vi "Large int-multiplty a and b.vi"(8 "error in (no error)":errorcluster, 10 "b = Large int (decimal)":string, 11 "a = Large int (decimal)":string) -> (0 "error out":errorcluster, 2 "T = the inputs are integers (contain only digits)":bool, 3 "c = a x b":string)   [LabVIEW 2021, in "Numeric Utilities.lvlib"]
uses:
  Numeric Utilities.lvlib
panel:
  out "longer integer":string
  out "shorter integer":string
  out "Loop iteration":i32
  # "Development\ncontrols/indicators useful for development and testing, but which are not outputs of the VI"
  # "Input\nInputs to the VI"
  # "Output\nOutputs of the VI"
  # "Description\n\nBlank VI with error handling case. \n\nSummarize the use of this VI in this space."
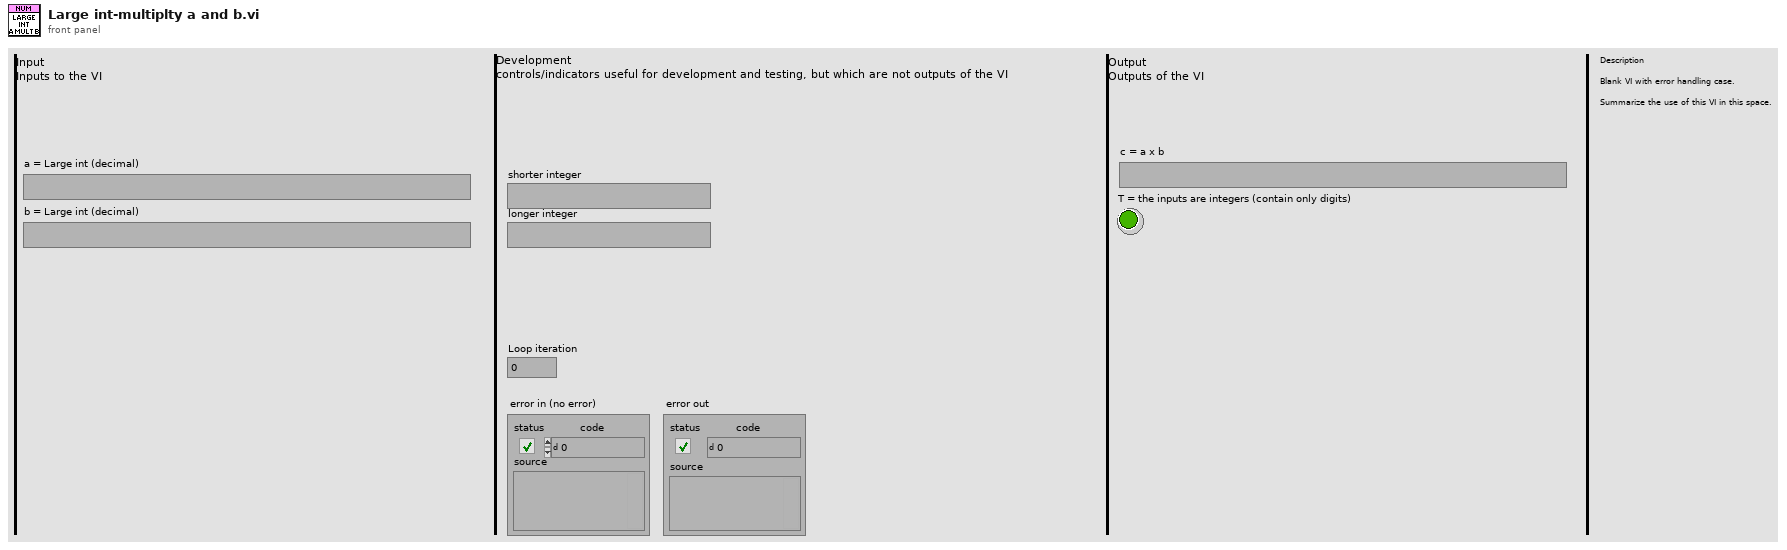
[diagram p1: front panel]
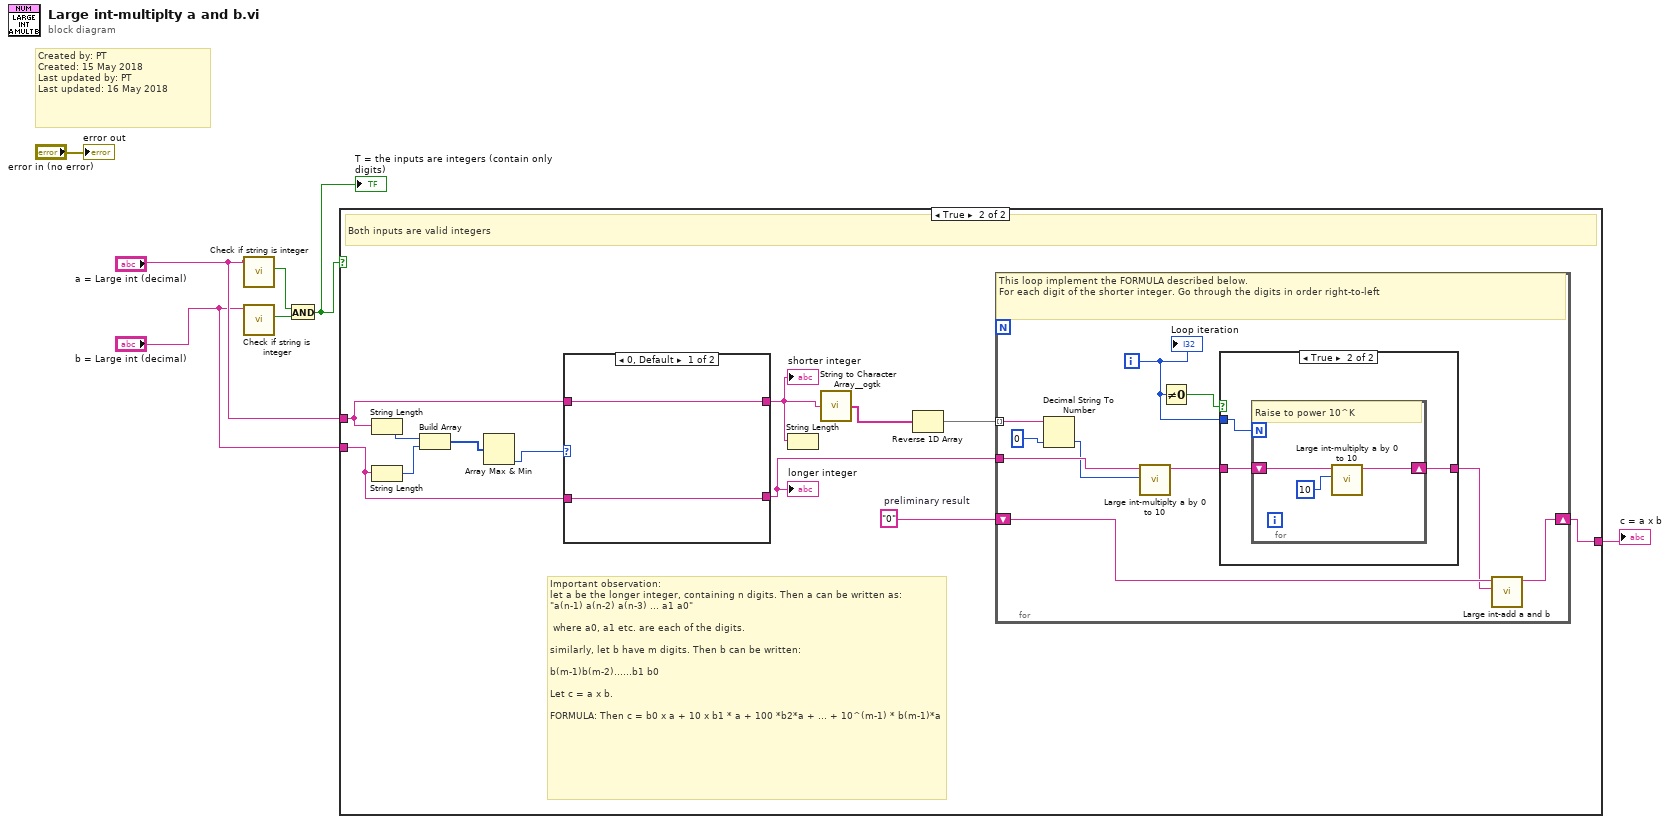
[diagram p0: block diagram]
diagram:
  # "Created by: PT\nCreated: 15 May 2018\nLast updated by: PT\nLast updated: 16 May 2018"
  n1 = call "Check if string is integer.vi"("string in"="a = Large int (decimal)") -> ("T = string contains an integer"=w3:bool)  [unwired: 8 in, 2 out]
  n2 = call "Check if string is integer.vi"("string in"="b = Large int (decimal)") -> ("T = string contains an integer"=w4:bool)  [unwired: 8 in, 2 out]
  n3 = And(x=w3, y=w4) -> (x .and. y?=w5:bool)
  "T = the inputs are integers (contain only digits)" <- w5
  n4 = case shown="True" w5 {
    tunnel: "a = Large int (decimal)" -> [_ w15]
    tunnel: [_ w9] -> w6
    tunnel: "b = Large int (decimal)" -> [_ w14]
    frame False {
      # "One or both inputs are not integers"
    }
    frame True {
      w19 = "0"  # preliminary result
      # "Important observation:\nlet a be the longer integer, containing n digits. Then a can be written as:\n\"a(n-1) a(n-2) a(n-3) ... a1 a0\"\n\n where a0, a1 etc. are each of the digits.\n\nsimilarly, let b have m digits. Then b can be written:\n\nb(m-1)b(m-2)......b1 b0\n\nLet c = a x b.\n\nFORMULA: Then c = b0 x a + 10 x b1 * a + 100 *b2*a + ... + 10^(m-1) * b(m-1)*a"
      # "Both inputs are valid integers"
      n5 = String Length(string=w15) -> (length=w18:i32)
      n6 = String Length(string=w14) -> (length=w17:i32)
      n7 = Build Array(w18, w17) -> (w16:i32[])
      n8 = Array Max & Min(array=w16) -> (min index (indices)=w8:i32)  [unwired: 3 out]
      n9 = case shown="0, Default" w8 {
        tunnel: w15 -> [w21 w23]
        tunnel: [w21 w22] -> w13
        tunnel: [w20 w23] -> w11
        tunnel: w14 -> [w20 w22]
        frame 0, Default {
        }
        frame 1 {
        }
      }
      "shorter integer" <- w13
      "longer integer" <- w11
      n10 = String Length(string=w13) -> ()  [unwired: 1 out]
      n11 = call <userlib>:"String to Character Array__ogtk.vi"("Input String"=w13) -> ("Character Array"=w12:string[])
      n12 = Reverse 1D Array(array=w12) -> (reversed array=w10:string[])
      n13 = for {
        tunnel: w10 -> [w32] mode=indexing
        shift-right: [w24] -> w9
        shift-left: w19 -> [w26]
        tunnel: w11 -> [w33]
        i -> [w27]
        # "This loop implement the FORMULA described below.\nFor each digit of the shorter integer. Go through the digits in order right-to-left"
        n14 = Decimal String To Number(string=w32, default (0L)=u32 0) -> (number=w31:u32)  [unwired: 1 in, 1 out]
        n15 = call "Large int-multiplty a by 0 to 10.vi"("b (0 to 10 inclusive)"=w31, "a = Large int (decimal)"=w33) -> ("c = a x b"=w28:string)  [unwired: 7 in, 2 out]
        n16 = Not Equal To 0?(x=w27) -> (x != 0?=w29:bool)
        n17 = case shown="True" w29 {
          tunnel: w28 -> [w34 w36]
          tunnel: [w34 w35] -> w25
          tunnel: w27 -> [_ w37]
          frame False {
            # "Least significant digit. 10^0 = 1"
          }
          frame True {
            n18 = for {
              N: w37 -> [_]
              shift-right: [w38] -> w35
              shift-left: w36 -> [w40]
              # "Raise to power 10^K"
              n19 = call "Large int-multiplty a by 0 to 10.vi"("b (0 to 10 inclusive)"=u32 10, "a = Large int (decimal)"=w40) -> ("c = a x b"=w38:string)  [unwired: 7 in, 2 out]
            }
          }
        }
        n20 = call "Large int-add a and b.vi"("b = Large int (decimal)"=w25, "a = Large int (decimal)"=w26) -> ("c = a x b"=w24:string)  [unwired: 7 in, 2 out]
        "Loop iteration" <- w27
      }
    }
  }
  "c = a x b" <- w6
  "error out" <- "error in (no error)"
